vi "GetStageAxesStatus (SubVI).vi"(0 ".NET Refnum in - Device":refnum<k24>, 2 "Axes Names":string[](array[string])=["X", "Y", "Z"], 3 "error in (no error)":errorcluster) -> (1 "Homed":bool, 4 "Axis enabled":cluster{"X":bool, "Y ":bool, "Z":bool}, 5 "Moving":bool, 6 ".NET Refnum out  - Device":refnum<k24>, 7 "Current stage position":T2, 8 "Current monitoring":T1, 9 "Stage position error":T2, 10 "error out":errorcluster)   [LabVIEW 2016]
doc: "Returns the Aerotech XYZ stage's current position per axis, or as a cluster with elements X position, Y position, and Z position. The units reflect those of the XYZ stage, so all the lengths are in mm. \n\nBuilt on top of the Aerotech .NET Libraries."
uses:
  C:/Users/Aerotech/Documents/BNLStaveAssembly-blueprint/Bin/Aerotech.A3200.dll
  BNLStaveAssembly-blueprint/Bin/Aerotech.A3200.dll
  AerotechLibraries/Status/AxisDiagPacket.ctl
panel:
  out "Axes":T3[](array[typedef])
  # "RETRIEVES THE PROPERTIES OF THE XYZ STAGE AXES"
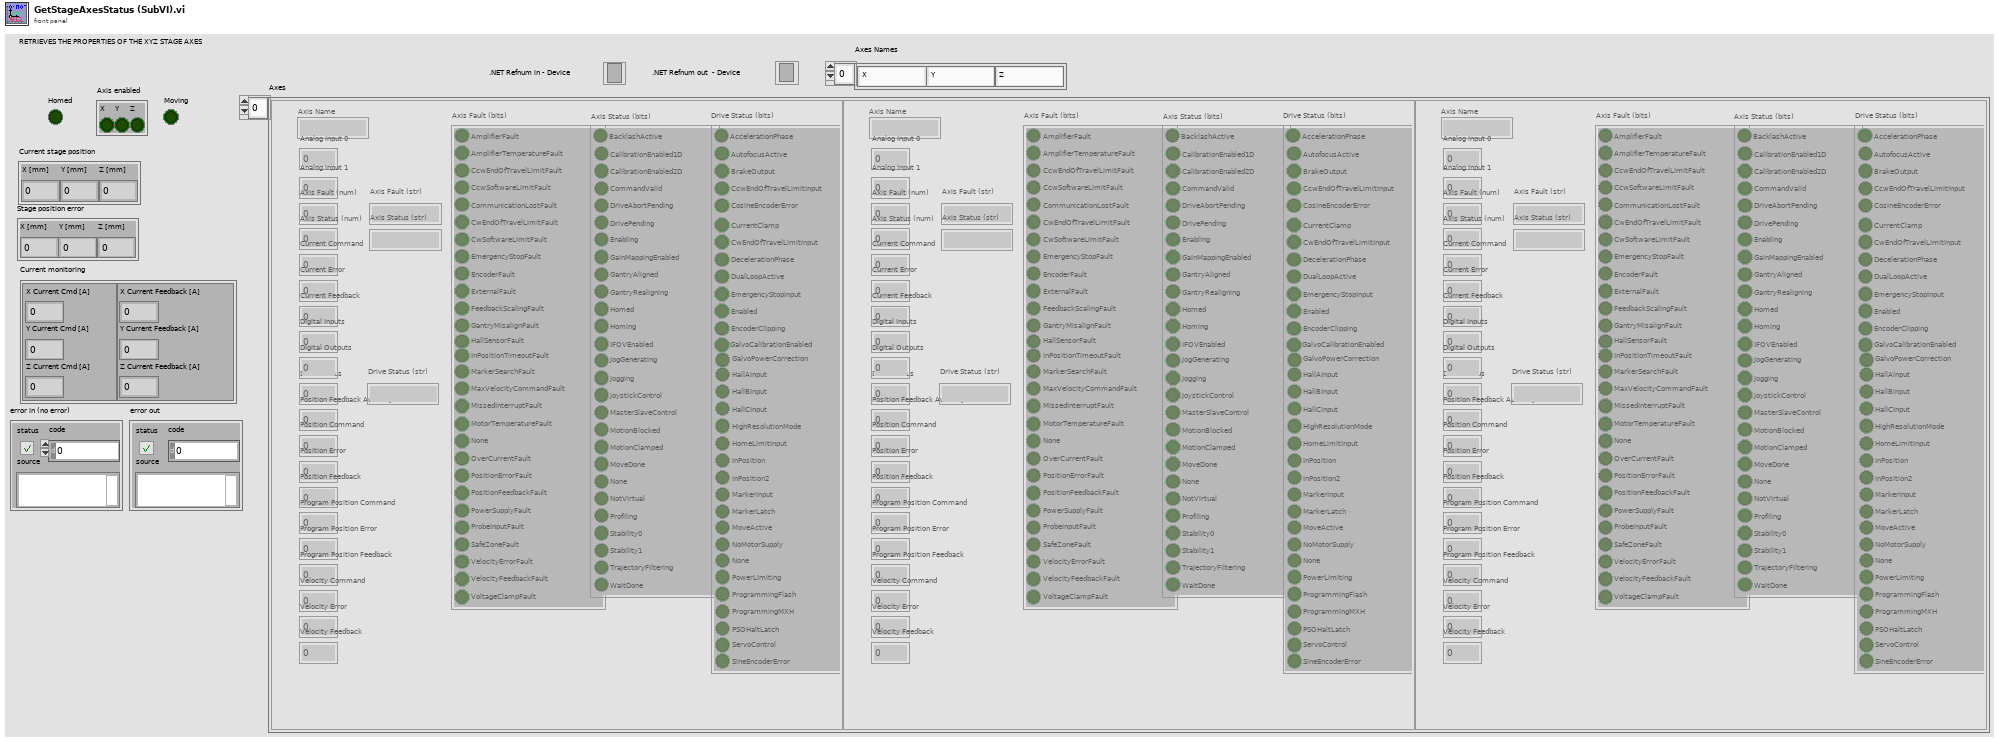
[diagram p1: front panel]
types:
  T1 = cluster{cluster{"X Current Cmd [A]":sgl, "Y Current Cmd [A]":sgl, "Z Current Cmd [A]":sgl}, cluster{"X Current Feedback [A]":sgl, "Y Current Feedback [A]":sgl, "Z Current Feedback [A]":sgl}}
  T2 = cluster{"X [mm]":dbl, "Y [mm]":dbl, "Z [mm]":dbl}
  T3 = typedef "AxisDiagPacket.ctl" = cluster{"Axis Name":string, "Analog Input 0":dbl, "Analog Input 1":dbl, "Axis Fault (num)":i32, "Axis Fault (str)":string, "Axis Fault (bits)":cluster{"AmplifierFault":bool, "AmplifierTemperatureFault":bool, "CcwEndOfTravelLimitFault":bool, "CcwSoftwareLimitFault":bool, "CommunicationLostFault":bool, "CwEndOfTravelLimitFault":bool, "CwSoftwareLimitFault":bool, "EmergencyStopFault":bool, "EncoderFault":bool, "ExternalFault":bool, "FeedbackScalingFault":bool, "GantryMisalignFault ":bool, "HallSensorFault":bool, "InPositionTimeoutFault":bool, "MarkerSearchFault":bool, "MaxVelocityCommandFault":bool, "MissedInterruptFault":bool, "MotorTemperatureFault":bool, "None":bool, "OverCurrentFault":bool, "PositionErrorFault":bool, "PositionFeedbackFault":bool, "PowerSupplyFault":bool, "ProbeInputFault":bool, "SafeZoneFault":bool, "VelocityErrorFault":bool, "VelocityFeedbackFault":bool, "VoltageClampFault":bool}, "Axis Status (num)":i32, "Axis Status (str)":string, "Axis Status (bits)":cluster{"BacklashActive":bool, "CalibrationEnabled1D":bool, "CalibrationEnabled2D":bool, "CommandValid":bool, "DriveAbortPending":bool, "DrivePending":bool, "Enabling":bool, "GainMappingEnabled":bool, "GantryAligned":bool, "GantryRealigning":bool, "Homed":bool, "Homing":bool, "IFOVEnabled":bool, "JogGenerating":bool, "Jogging":bool, "JoystickControl":bool, "MasterSlaveControl":bool, "MotionBlocked":bool, "MotionClamped":bool, "MoveDone":bool, "None":bool, "NotVirtual":bool, "Profiling":bool, "Stability0":bool, "Stability1":bool, "TrajectoryFiltering":bool, "WaitDone":bool}, "Current Command":sgl, "Current Error":sgl, "Current Feedback":sgl, "Digital Inputs":i32, "Digital Outputs":i32, "Drive Status":i32, "Drive Status (str)":string, "Drive Status (bits)":cluster{"AccelerationPhase":bool, "AutofocusActive":bool, "BrakeOutput":bool, "CcwEndOfTravelLimitInput":bool, "CosineEncoderError":bool, "CurrentClamp":bool, "CwEndOfTravelLimitInput":bool, "DecelerationPhase":bool, "DualLoopActive":bool, "EmergencyStopInput":bool, "Enabled":bool, "EncoderClipping":bool, "GalvoCalibrationEnabled":bool, "GalvoPowerCorrection":bool, "HallAInput":bool, "HallBInput":bool, "HallCInput":bool, "HighResolutionMode":bool, "HomeLimitInput":bool, "InPosition":bool, "InPosition2":bool, "MarkerInput":bool, "MarkerLatch":bool, "MoveActive":bool, "NoMotorSupply":bool, "None":bool, "PowerLimiting":bool, "ProgrammingFlash":bool, "ProgrammingMXH":bool, "PSOHaltLatch":bool, "ServoControl":bool, "SineEncoderError":bool}, "Position Feedback Auxiliary":dbl, "Position Command":dbl, "Position Error":dbl, "Position Feedback":dbl, "Program Position Command":dbl, "Program Position Error":dbl, "Program Position Feedback":dbl, "Velocity Command":dbl, "Velocity Error":dbl, "Velocity Feedback":dbl}
  T4 = typedef "ControllerDiagPacket.ctl" = cluster{"Number of Diag Packets":i32, "Axes":T3[], "error":errorcluster}
  T5 = cluster{"Axes Names[0]":string, "Axes Names[1]":string, "Axes Names[2]":string, "Axes Names[3]":string, "Axes Names[4]":string, "Axes Names[5]":string, "Axes Names[6]":string, "Axes Names[7]":string, "Axes Names[8]":string}
  T6 = cluster{"Program Position Feedback":dbl, "Program Position Feedback":dbl, "Program Position Feedback":dbl}
  T7 = cluster{"Program Position Error":dbl, "Program Position Error":dbl, "Program Position Error":dbl}
  T8 = cluster{"Current Command":sgl, "Current Command":sgl, "Current Command":sgl}
  T9 = cluster{"Current Feedback":sgl, "Current Feedback":sgl, "Current Feedback":sgl}
  T10 = cluster{"Enabled":bool, "Enabled":bool, "Enabled":bool}
  T11 = cluster{cluster{"Current Command":sgl, "Current Command":sgl, "Current Command":sgl}, cluster{"Current Feedback":sgl, "Current Feedback":sgl, "Current Feedback":sgl}}
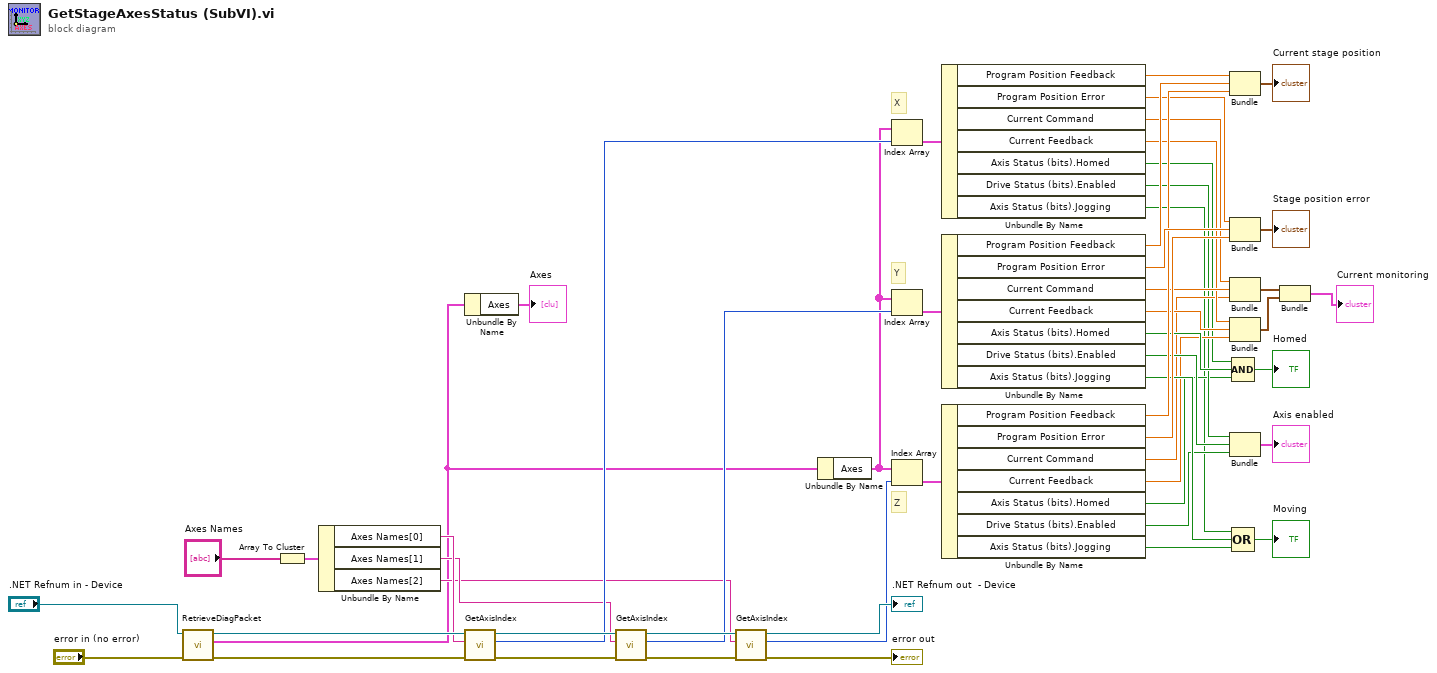
[diagram p0: block diagram]
diagram:
  # "Y"
  # "Z"
  # "X"
  n1 = call "RetrieveDiagPacket.vi"("error in (no error)"="error in (no error)", "Controller In"=".NET Refnum in - Device") -> ("error out"=w40:errorcluster, "ControllerDiagPacket"=w32:T4, "Controller Out"=w45:refnum<k24>)  [unwired: 7 in]
  n2 = Array To Cluster(array="Axes Names") -> (cluster=w38:T5)
  n3 = Unbundle By Name(w38) -> ("Axes Names[0]"=w37:string, "Axes Names[1]"=w36:string, "Axes Names[2]"=w35:string)
  n4 = Unbundle By Name(w32) -> ("Axes"=→"Axes":T3[])
  n5 = call "GetAxisIndex.vi"("error in (no error)"=w40, "axis name"=w37, "controller in"=w45) -> ("error out"=w44:errorcluster, "axis index"=w41:i32, "controller out"=w46:refnum<k24>)  [unwired: 6 in]
  n6 = call "GetAxisIndex.vi"("error in (no error)"=w44, "axis name"=w36, "controller in"=w46) -> ("error out"=w49:errorcluster, "axis index"=w43:i32, "controller out"=w52:refnum<k24>)  [unwired: 6 in]
  n7 = call "GetAxisIndex.vi"("error in (no error)"=w49, "axis name"=w35, "controller in"=w52) -> ("error out"=→"error out":errorcluster, "axis index"=w51:i32, "controller out"=→".NET Refnum out  - Device":refnum<k24>)  [unwired: 6 in]
  n8 = Unbundle By Name(w32) -> ("Axes"=w31:T3[])
  n9 = Index Array(array=w31, index=w41) -> (element=w29:T3)
  n10 = Index Array(array=w31, index=w43) -> (element=w42:T3)
  n11 = Index Array(array=w31, index=w51) -> (element=w7:T3)
  n12 = Unbundle By Name(w29) -> ("Program Position Feedback"=w28:dbl, "Program Position Error"=w24:dbl, "Current Command"=w16:sgl, "Current Feedback"=w17:sgl, "Axis Status (bits).Homed"=w13:bool, "Drive Status (bits).Enabled"=w11:bool, "Axis Status (bits).Jogging"=w1:bool)
  n13 = Unbundle By Name(w42) -> ("Program Position Feedback"=w34:dbl, "Program Position Error"=w30:dbl, "Current Command"=w22:sgl, "Current Feedback"=w21:sgl, "Axis Status (bits).Homed"=w20:bool, "Drive Status (bits).Enabled"=w18:bool, "Axis Status (bits).Jogging"=w19:bool)
  n14 = Unbundle By Name(w7) -> ("Program Position Feedback"=w27:dbl, "Program Position Error"=w26:dbl, "Current Command"=w14:sgl, "Current Feedback"=w15:sgl, "Axis Status (bits).Homed"=w2:bool, "Drive Status (bits).Enabled"=w10:bool, "Axis Status (bits).Jogging"=w3:bool)
  n15 = Bundle("Program Position Feedback"=w28, "Program Position Feedback"=w34, "Program Position Feedback"=w27) -> (→"Current stage position":T6)  [unwired: 1 in]
  n16 = Bundle("Program Position Error"=w24, "Program Position Error"=w30, "Program Position Error"=w26) -> (→"Stage position error":T7)  [unwired: 1 in]
  n17 = Bundle("Current Command"=w16, "Current Command"=w22, "Current Command"=w14) -> (w6:T8)  [unwired: 1 in]
  n18 = Bundle("Current Feedback"=w17, "Current Feedback"=w21, "Current Feedback"=w15) -> (w5:T9)  [unwired: 1 in]
  n19 = Bundle("Enabled"=w11, "Enabled"=w18, "Enabled"=w10) -> (→"Axis enabled":T10)  [unwired: 1 in]
  n20 = Compound Arithmetic op=AND(w13, w20, w2) -> (→"Homed":bool)
  n21 = Compound Arithmetic op=OR(w1, w19, w3) -> (→"Moving":bool)
  n22 = Bundle(w6, w5) -> (→"Current monitoring":T11)  [unwired: 1 in]
